vi "Init.vi"(0 "address":string="192.168.1.100", 1 "Name":string="NVM 1", 2 "ParentName":string="STAND", 5 "addres":u16=1, 7 "SV_Publisher":refnum<class "SV_Publisher.lvclass">, 11 "error in (no error)":errorcluster, 12 "ConfigInterface":refnum<class "ConfigInterface.lvclass">, 14 "Logger":refnum<class "Logger.lvclass">) -> (4 "NeedleValve out":refnum<class "NeedleValve.lvclass">, 15 "error out":errorcluster)   [LabVIEW 2019, in "NeedleValve.lvclass"]
uses:
  NeedleValve.lvclass
  C:/Users/H4001/Documents/GitHub/H4000/src/Proccess_class/Proccess.lvclass
  C:/Users/H4001/Documents/GitHub/H4000/src/Device_class/Device.lvclass
  ConfigInterface_class/ConfigInterface.lvclass
  Logger_class/Logger.lvclass
  SV_Puplisher_class/SV_Publisher.lvclass
  modbus engine custom/MB_ENGINE_class/MB_ENGINE.lvclass
  MessageAMC_class/MessageAMC.lvclass
  C:/Users/H4001/Documents/GitHub/H4000/src/MessageInterface_class/MessageInterface.lvclass
  modbus engine custom/MB_ENGINE_class/Switch Rule and Polarity.ctl
  modbus engine custom/MB_ENGINE_class/cmd enum.ctl
  TypeDef/Needle Valve State.ctl
  NeedleValve.lvclass/NeedleValve.ctl
  <vilib>/NI/Modbus Library/API/Wrapper/Create TCP Master.vi
  <vilib>/NI/Modbus Library/API/Wrapper/API Main.lvlib
  Proccess_class/Proccess.lvclass
  Device_class/Device.lvclass
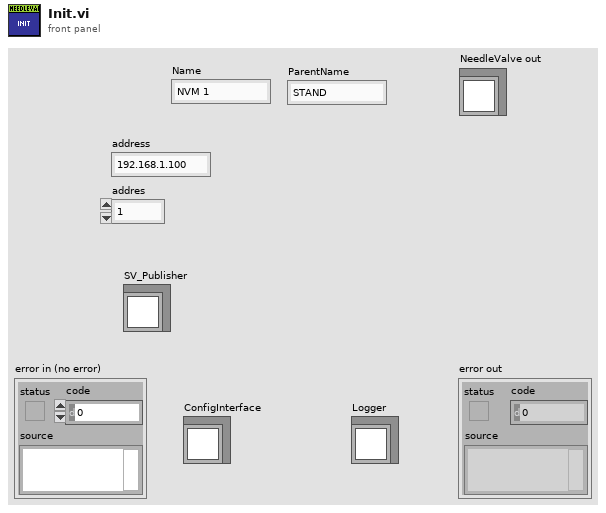
[diagram p1: front panel]
types:
  T1 = typedef "Needle Valve State.ctl" = enum16{"IDLE", "OPENING", "CLOSING", "STOP"}
  T2 = typedef "MB_ENGINE.lvclass/Switch Rule and Polarity.ctl" = cluster{"Switch Rule":u8, "Polarity, F - NO, T - NC":bool}
  T3 = typedef "MB_ENGINE.lvclass/cmd enum.ctl" = u16
  T4 = typedef "MB_ENGINE.lvclass/Settings.ctl" = cluster{"ACC Steps Per Sec^2":u16, "DEC Steps Per Sec^2":u16, "Min Velosity Step Per Sec":u16, "Max Velosity Step Per Sec":u16, "MicroStep":u16}
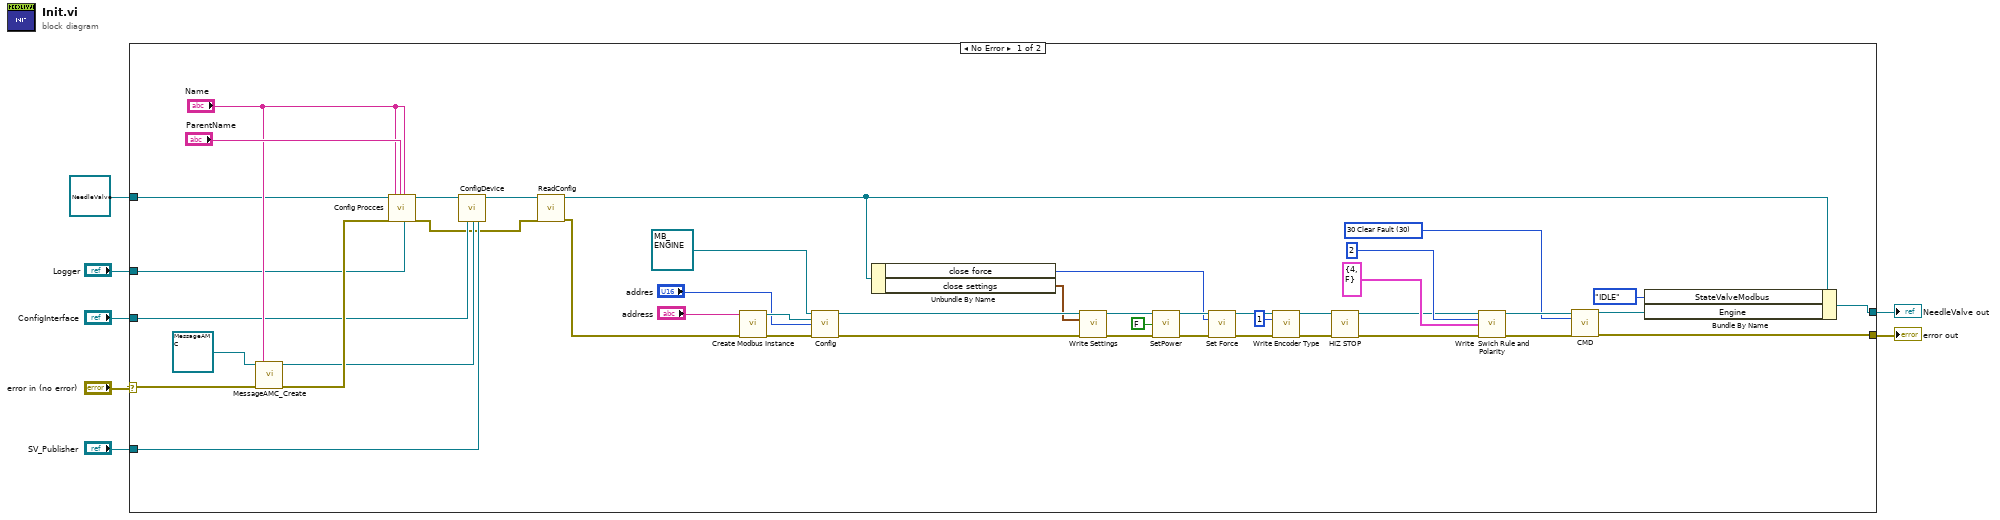
[diagram p0: block diagram]
diagram:
  n1 = case shown="No Error" "error in (no error)" {
    selector: "error in (no error)" -> [w21 w54]
    tunnel: [w15 w54] -> w6
    tunnel: [w16 w53] -> w4
    tunnel: refnum<class "NeedleValve.lvclass"> refnum ("NeedleValve in") -> [w22 w53]
    tunnel: "ConfigInterface" -> [w13 _]
    tunnel: "Logger" -> [w23 _]
    tunnel: "SV_Publisher" -> [w12 _]
    frame No Error {
      w26 = T3 30 items=["0 Idle"=0, "1 GoTo Absolute Position"=1, "2 GoTo Relative"=2, "10 GoTo Home Position"=10, "11 Set Home Position"=11, "12 Set FindHome Mode"=12, "13 Reset FindHome Mode"=13, "14 Get FindHome State"=14, "20 Hard Stop"=20, "21 HiZ Stop"=21, "22 Soft Stop"=22, "30 Clear Fault"=30, "40 Encoder Set Home"=40, "70 Driver Init"=70] ("cmd to write")
      n2 = call "MessageAMC_Create.vi"("reference in"=refnum<class "MessageAMC.lvclass"> refnum, "error in (no error)"=w21, "message queue name"="Name") -> ("amc"=w11:refnum<class "MessageAMC.lvclass">, "error out"=w34:errorcluster)  [unwired: 15 in]
      n3 = call "Config Procces.vi"("reference in"=w22, "error in (no error)"=w34, "Name"="Name", "ParentName"="ParentName", "Description"="Name", "Logger"=w23) -> ("reference out"=w14:refnum<class "NeedleValve.lvclass">, "error out"=w9:errorcluster)  [unwired: 12 in]
      n4 = call "ConfigDevice.vi"("Device in"=w14, "ConfigInterface"=w13, "MessageInterface"=w11, "SV_Publisher"=w12) -> ("Device out"=w10:refnum<class "NeedleValve.lvclass">)  [unwired: 11 in]
      n5 = call-dynamic "ReadConfig.vi"("reference in"=w10, "error in (no error)"=w9) -> ("reference out"=w19:refnum<class "NeedleValve.lvclass">, "error out"=w20:errorcluster)  [unwired: 12 in]
      n6 = call-poly <vilib>:"Create Modbus Instance.vi"("error in"=w20, "address"="address") -> ("error out"=w44:errorcluster, "TCP master instance"=w43:refnum<class "Modbus Master.lvclass">)  [unwired: 8 in]
      n7 = call-dynamic "Config.vi"("class data in"=refnum<class "MB_ENGINE.lvclass"> refnum ("MB_ENGINE"), "modbus"=w43, "addres"="addres", "error in (no error)"=w44) -> ("class data out"=w45:refnum<class "MB_ENGINE.lvclass">, "error out"=w46:errorcluster)  [unwired: 10 in]
      n8 = Unbundle By Name(w19) -> ("close force"=w18:u16, "close settings"=w17:T4)
      n9 = call "Write Settings.vi"("class data in"=w45, "cluster"=w17, "error in (no error)"=w46) -> ("class data out"=w47:refnum<class "MB_ENGINE.lvclass">, "error out"=w52:errorcluster)  [unwired: 11 in]
      n10 = call "SetPower.vi"("class data in"=w47, "On"=FALSE, "error in (no error)"=w52) -> ("class data out"=w48:refnum<class "MB_ENGINE.lvclass">, "error out"=w49:errorcluster)  [unwired: 11 in]
      n11 = call "Set Force.vi"("class data in"=w48, "percent"=w18, "error in (no error)"=w49) -> ("class data out"=w50:refnum<class "MB_ENGINE.lvclass">, "error out"=w51:errorcluster)  [unwired: 11 in]
      n12 = call-dynamic "Write Encoder Type.vi"("class data in"=w50, "U16"=u16 1, "error in (no error)"=w51) -> ("class data out"=w33:refnum<class "MB_ENGINE.lvclass">, "error out"=w32:errorcluster)  [unwired: 11 in]
      n13 = call-dynamic "HIZ STOP.vi"("class data in"=w33, "error in (no error)"=w32) -> ("class data out"=w29:refnum<class "MB_ENGINE.lvclass">, "error out"=w28:errorcluster)  [unwired: 12 in]
      n14 = call-dynamic "Write  Swich Rule and Polarity.vi"("class data in"=w29, "SW"=u16 2, "Switch Rule and Polarity"=T2 {"Switch Rule"=4, "Polarity, F - NO, T - NC"=FALSE}, "error in (no error)"=w28) -> ("class data out"=w27:refnum<class "MB_ENGINE.lvclass">, "error out"=w25:errorcluster)  [unwired: 10 in]
      n15 = call "CMD.vi"("class data in"=w27, "cmd to write"=w26, "error in (no error)"=w25) -> ("class data out"=w24:refnum<class "MB_ENGINE.lvclass">, "error out"=w15:errorcluster)  [unwired: 11 in]
      n16 = Bundle By Name(cluster=w19, "StateValveModbus"=Needle_Valve_State."IDLE" ("Needle Valve Data.StateValveModbus"), "Engine"=w24) -> (w16:refnum<class "NeedleValve.lvclass">)
    }
    frame Error {
    }
  }
  "error out" <- w6
  "NeedleValve out" <- w4
